vi "Transform Position.vi"(2 "error in (no error)":errorcluster, 3 "Car.lvclass":refnum<class "Car.lvclass">, 4 "Sensor.lvclass":refnum<class "Sensor.lvclass">) -> (0 "error out":errorcluster, 1 "Sensor.lvclass 2":refnum<class "Sensor.lvclass">)   [LabVIEW 2015, in "Sensor.lvclass"]
uses:
  Sensor.lvclass
  Car.lvclass
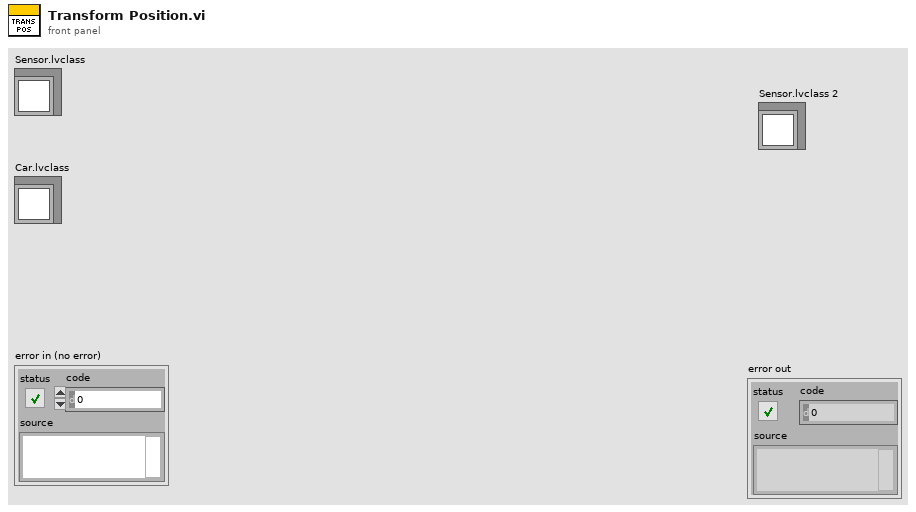
[diagram p1: front panel]
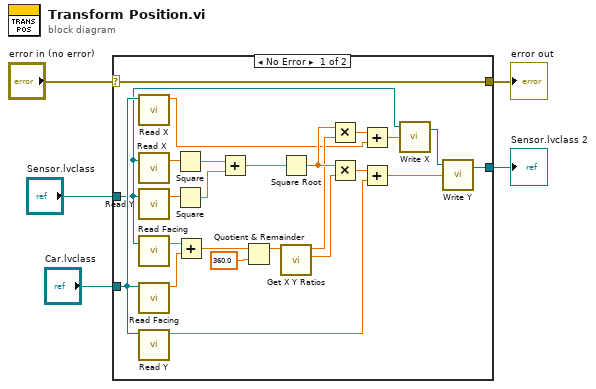
[diagram p0: block diagram]
diagram:
  n1 = case shown="No Error" "error in (no error)" {
    selector: "error in (no error)" -> [w29 w30]
    tunnel: [w29 w30] -> w4
    tunnel: [w8 w31] -> w3
    tunnel: "Sensor.lvclass" -> [w12 w31]
    tunnel: "Car.lvclass" -> [w15 _]
    frame No Error {
      n2 = call "Read X.vi"("Car.lvclass"=w15) -> ("X"=w6:dbl)  [unwired: 9 in, 1 out]
      n3 = call "Read X.vi"("Sensor.lvclass"=w12) -> ("X"=w28:dbl)  [unwired: 1 in, 1 out]
      n4 = call "Read Y.vi"("Sensor.lvclass"=w12) -> ("Y"=w27:dbl)  [unwired: 1 in, 1 out]
      n5 = call "Read Facing.vi"("Sensor.lvclass"=w12) -> ("Facing"=w23:dbl)  [unwired: 1 in, 1 out]
      n6 = call "Read Facing.vi"("Car.lvclass"=w15) -> ("Facing"=w22:dbl)  [unwired: 9 in, 1 out]
      n7 = call "Read Y.vi"("Car.lvclass"=w15) -> ("Y"=w7:dbl)  [unwired: 9 in, 1 out]
      n8 = Square(x=w28) -> (x^2=w26:dbl)
      n9 = Square(x=w27) -> (x^2=w25:dbl)
      n10 = Add(x=w23, y=w22) -> (x+y=w21:dbl)
      n11 = Add(x=w26, y=w25) -> (x+y=w24:dbl)
      n12 = Quotient & Remainder(x=w21, y=360.0) -> (x-y*floor(x/y)=w19:dbl)  [unwired: 1 out]
      n13 = Square Root(x=w24) -> (sqrt(x)=w18:dbl)
      n14 = call "Get X Y Ratios.vi"("Facing"=w19) -> ("Y Ratio"=w16:dbl, "X Ratio"=w17:dbl)  [unwired: 9 in]
      n15 = Multiply(x=w18, y=w17) -> (x*y=w14:dbl)
      n16 = Multiply(x=w18, y=w16) -> (x*y=w13:dbl)
      n17 = Add(x=w14, y=w6) -> (x+y=w9:dbl)
      n18 = Add(x=w13, y=w7) -> (x+y=w10:dbl)
      n19 = call "Write X.vi"("X"=w9, "Sensor In"=w12) -> ("Sensor Out"=w11:refnum<class "Sensor.lvclass">)  [unwired: 1 in, 1 out]
      n20 = call "Write Y.vi"("Y"=w10, "Sensor In"=w11) -> ("Sensor Out"=w8:refnum<class "Sensor.lvclass">)  [unwired: 1 in, 1 out]
    }
    frame Error {
    }
  }
  "error out" <- w4
  "Sensor.lvclass 2" <- w3
